vi "Initialize Joystick.vi"(8 "error in (no error)":errorcluster, 10 "Joystick":refnum<class "Joystick.lvclass">, 11 "Driver in":refnum<class "Driver.lvclass">) -> (0 "error out":errorcluster, 3 "Driver out":refnum<class "Driver.lvclass">)   [LabVIEW 2014, in "Driver.lvlib" / "Driver.lvclass"]
uses:
  Driver.lvclass
  Joystick/Joystick Class/Joystick.lvclass
  Driver.lvclass/Driver.ctl
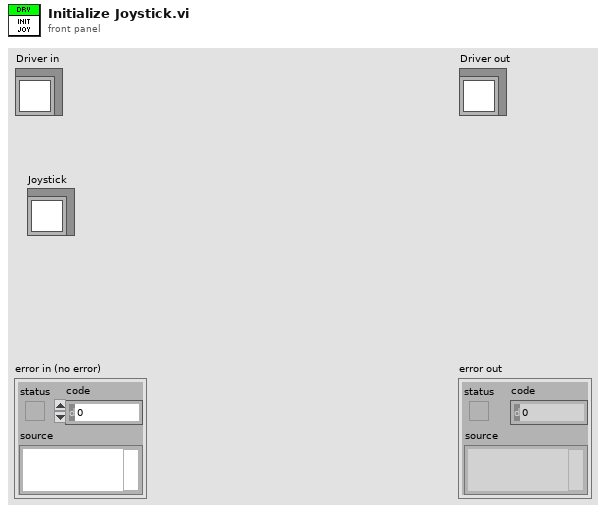
[diagram p1: front panel]
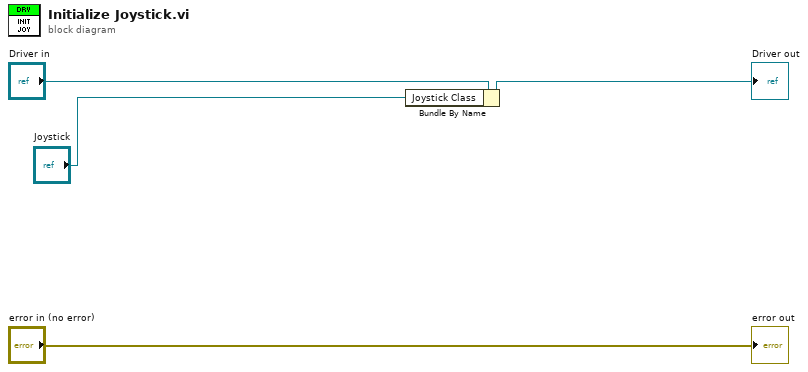
[diagram p0: block diagram]
diagram:
  n1 = Bundle By Name(cluster="Driver in", "Joystick Class"="Joystick") -> (→"Driver out":refnum<class "Driver.lvclass">)
  "error out" <- "error in (no error)"
